vi "getPositionAllAxis.vi"(8 "error":errorcluster, 11 "connection ID":refnum<k5>) -> (0 "error out":errorcluster, 2 "AllAxisPositions_um":T1, 3 "connection ID out":refnum<k5>)   [LabVIEW 2016, in "AMC_VIs.lvlib"]
doc: "This function returns the position of all three axes in um\nIf there is no positioner on one axis, it returns zero instead\nMove function\nInputs:\n none\nOutputs:\n err\n pos_um_x position of the x-axis in um\n pos_um_y position of the y-axis in um\n pos_um_z position of the z-axis in um"
uses:
  AMC_VIs.lvlib
panel:
  out "JSON-response":string="{\"jsonrpc\":\"2.0\",\"method\":\"\",\"params\":[5,1.245,true,\"name\"],\"id\":\"1\"}"
  out "JSON request":string
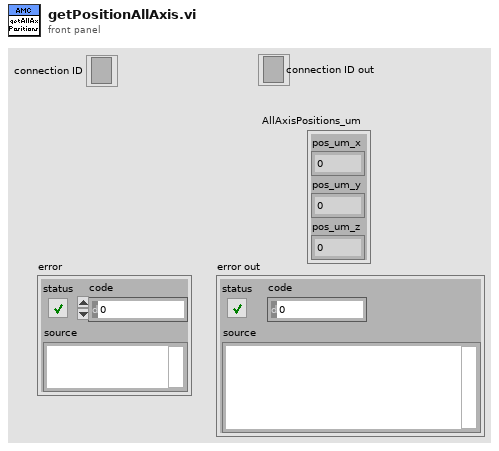
[diagram p1: front panel]
types:
  T1 = cluster{"pos_um_x":dbl, "pos_um_y":dbl, "pos_um_z":dbl}
  T2 = cluster{"jsonrpc":string, "method":string, "params":i32[], "id":string, "api":string}
  T3 = cluster{"jsonrpc":string, "result":i32[], "id":string}
  T4 = enum16{"Standard", "Buffered", "CRLF", "Immediate"}
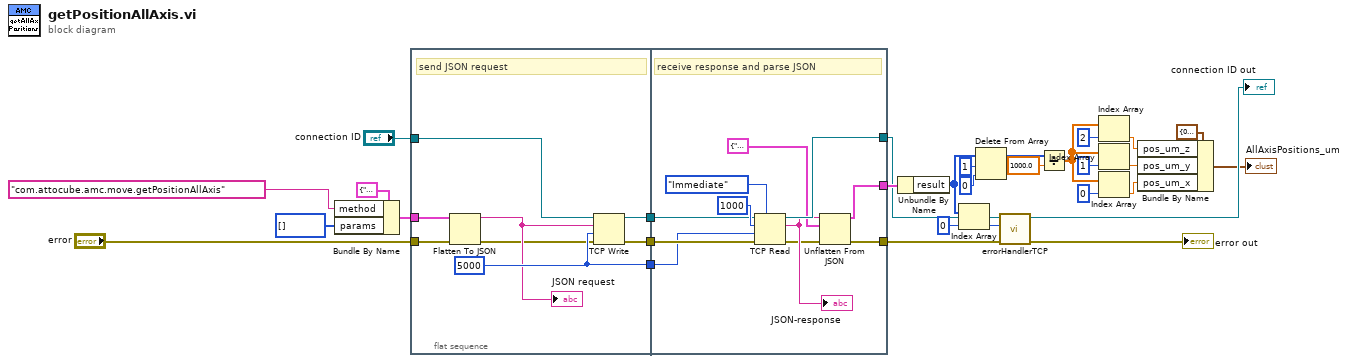
[diagram p0: block diagram]
diagram:
  n1 = Bundle By Name(cluster=T2 {"jsonrpc"="2.0", "method"="com.attocube.amc.res.setRESReadOutFreq", "params"=[0, 2712], "id"="1", "api"="2"} ("InputParams 2"), "method"="com.attocube.amc.move.getPositionAllAxis", "params"=i32[] []) -> (w23:T2)
  n2 = flat-sequence {
    tunnel: "connection ID" -> [w38]
    tunnel: [w36] -> w30
    tunnel: [w37] -> w29
    tunnel: "error" -> [w32]
    tunnel: [w35] -> w28
    tunnel: w23 -> [w34]
    tunnel: [w45] -> w16
    tunnel: w30 -> [w47]
    tunnel: w29 -> [w46]
    tunnel: [w41] -> w19
    tunnel: w28 -> [w44]
    tunnel: [w40] -> w22
    frame #0 {
      w35 = 5000 ("timeout ms (25000)")
      # "send JSON request"
      n3 = Flatten To JSON(anything=w34, error in (no error)=w32) -> (JSON string=w33:string, 11:w31:errorcluster)  [unwired: 1 in]
      "JSON request" <- w33
      n4 = TCP Write(connection ID=w38, data in=w33, error in (no error)=w31, 9:w35) -> (connection ID out=w36:refnum<k5>, error out=w37:errorcluster)  [unwired: 1 out]
    }
    frame #1 {
      # "receive response and parse JSON"
      n5 = TCP Read(connection ID=w47, bytes to read=1000, error in (no error)=w46, 7:T4."Immediate" ("mode (standard)"), 9:w44) -> (connection ID out=w45:refnum<k5>, data out=w43:string, error out=w42:errorcluster)
      "JSON-response" <- w43
      n6 = Unflatten From JSON(JSON string=w43, type and defaults=T3 {"jsonrpc"="2.0", "result"=[0, 2712], "id"="1"} ("InputParams 2"), error in (no error)=w42) -> (value=w40:T3, error out=w41:errorcluster)  [unwired: 4 in]
    }
  }
  n7 = Unbundle By Name(w22) -> ("result"=w11:i32[])
  n8 = Index Array(array=w11, index=0) -> (element=w18:i32)
  n9 = Delete From Array(array=w11, length=1, index=0) -> (array with subset deleted=w8:i32[])  [unwired: 1 out]
  n10 = call "errorHandlerTCP.vi"("error in"=w19, "error number"=w18, "connection ID"=w16) -> ("error out"=→"error out":errorcluster, "connection ID"=→"connection ID out":refnum<k5>)  [unwired: 7 in]
  n11 = Divide(x=w8, y=1000.0) -> (x/y=w7:dbl[])
  n12 = Index Array(array=w7, index=2) -> (element=w3:dbl)
  n13 = Index Array(array=w7, index=1) -> (element=w4:dbl)
  n14 = Index Array(array=w7, index=0) -> (element=w5:dbl)
  n15 = Bundle By Name(cluster=T1 {"pos_um_x"=0.0, "pos_um_y"=0.0, "pos_um_z"=0.0}, "pos_um_z"=w3, "pos_um_y"=w4, "pos_um_x"=w5) -> (→"AllAxisPositions_um":T1)
